vi "Read Request With Reply Links.vi"(8 "error in (no error)":errorcluster, 11 "Dqmh Module in":refnum<class "Dqmh Module.lvclass">) -> (0 "error out":errorcluster, 2 "Request With Reply Links":T1[](array[typedef]), 3 "Dqmh Module out":refnum<class "Dqmh Module.lvclass">)   [LabVIEW 2021, in "TAF Proj Document Type.lvlib" / "Dqmh Module.lvclass"]
uses:
  <vilib>/Wovalab/AntiDoc/Document Type/Add-ons/LabVIEW TAF Project/Dqmh Module/Dqmh Module.lvclass
  <vilib>/Wovalab/AntiDoc/Document Type/Add-ons/LabVIEW TAF Project/Dqmh Module/Event Callers--cluster.ctl
  <vilib>/Wovalab/AntiDoc/Document Type/Add-ons/LabVIEW TAF Project/Dqmh Module/Dqmh Module.lvclass/Dqmh Module.ctl
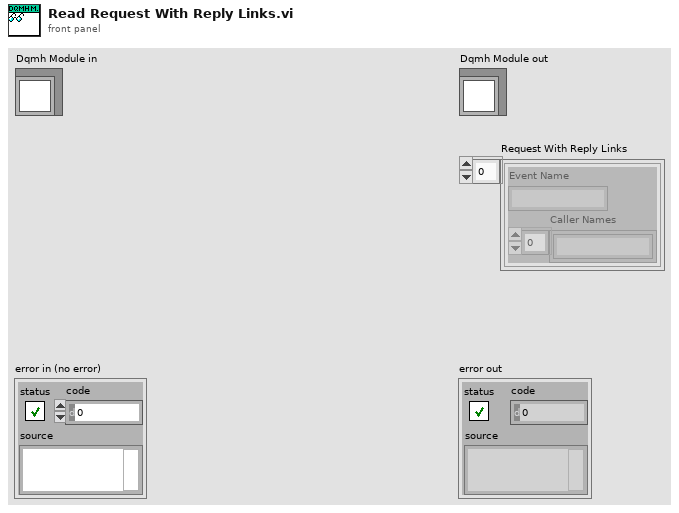
[diagram p1: front panel]
types:
  T1 = typedef "TAF Proj Document Type.lvlib/Dqmh Module.lvclass/Event Callers--cluster.ctl" = cluster{"Event Name":string, "Caller Names":string[]}
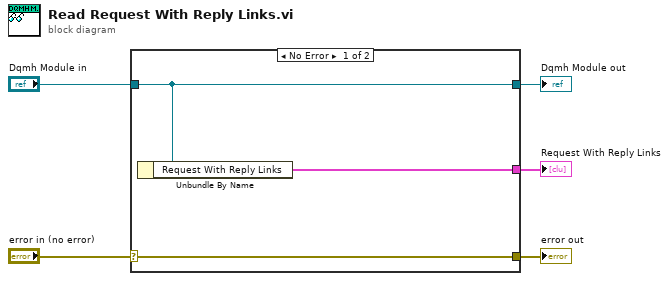
[diagram p0: block diagram]
diagram:
  n1 = case shown="No Error" "error in (no error)" {
    selector: "error in (no error)" -> [w8 w9]
    tunnel: [w8 w9] -> w4
    tunnel: [w7 w10] -> w2
    tunnel: "Dqmh Module in" -> [w7 w10]
    tunnel: [w6 _] -> w1
    frame No Error {
      n2 = Unbundle By Name(w7) -> ("Request With Reply Links"=w6:T1[])
    }
    frame Error {
    }
  }
  "error out" <- w4
  "Dqmh Module out" <- w2
  "Request With Reply Links" <- w1
